vi "Complete Request.vi"(4 "WebSocket Handler":refnum<class "WebSocket Handler.lvclass">, 9 "Complete Handler Map":T1, 11 "Processing In":refnum<class "Processing.lvclass">) -> (3 "HTTP Server.lvlib:Processing":refnum<class "Processing.lvclass">)   [LabVIEW 2020, in "HTTP Server.lvlib" / "Server.lvclass"]
uses:
  Server.lvclass
  Processing/Processing.lvclass
  Complete Handler Map.ctl
  Priority.ctl
  Complete Handler/Complete Handler.lvclass
  WebSocket Handler/WebSocket Handler.lvclass
  C:/dev/lv20CE/relink/lv-http-server/HTTP Server/Handler/Handler.lvclass
  C:/dev/lv20CE/relink/lv-http-server/HTTP Server/Complete Handler/Complete Handler.lvclass
  Processing Step.ctl
  Processing/Processing.lvclass/Processing.ctl
  Handler/Handler.lvclass
  Server.lvclass/Server.ctl
  Session/Session.lvclass
  HTTP Server.lvlib
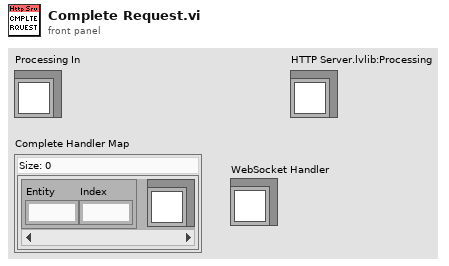
[diagram p1: front panel]
types:
  T1 = typedef "HTTP Server.lvlib/Complete Handler Map.ctl" = map{T2, refnum<class "Complete Handler.lvclass">}
  T2 = typedef "HTTP Server.lvlib/Priority.ctl" = cluster{"Entity":u16, "Index":u16}
  T3 = typedef "HTTP Server.lvlib/Processing Step.ctl" = enum16{"Connection", "Request", "Routing", "Controller Init", "Controller", "Response", "Complete", "Exception"}
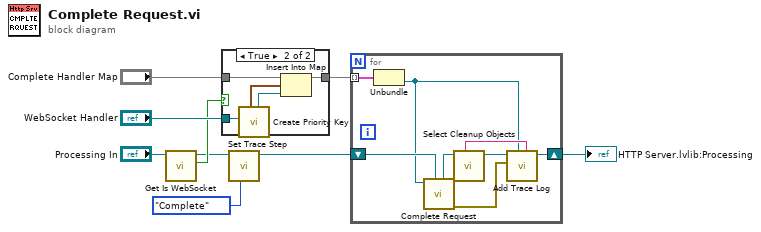
[diagram p0: block diagram]
diagram:
  n1 = call "Get Is WebSocket.vi"("Processing in"="Processing In") -> ("Is WebSocket"=w5:bool, "Processing out"=w4:refnum<class "Processing.lvclass">)  [unwired: 9 in]
  n2 = case shown="True" w5 {
    tunnel: "Complete Handler Map" -> [w10 w13]
    tunnel: "WebSocket Handler" -> [_ w11]
    tunnel: [w10 w12] -> w7
    frame False {
    }
    frame True {
      n3 = call "Create Priority Key.vi"("Handler In"=w11) -> ("Handler"=w14:refnum<class "WebSocket Handler.lvclass">, "Priority Key"=w15:T2)  [unwired: 8 in, 1 out]
      n4 = Insert Into Map(map in=w13, key=w15, value=w14) -> (map out=w12:T1)  [unwired: 2 out]
    }
  }
  n5 = call "Set Trace Step.vi"("Processing Step"=Processing_Step."Complete", "Processing in"=w4) -> ("Processing out"=w3:refnum<class "Processing.lvclass">)  [unwired: 9 in]
  n6 = for {
    tunnel: w7 -> [w23] mode=indexing
    shift-right: [w16] -> w2
    shift-left: w3 -> [w22]
    n7 = Unbundle(w23) -> ("Handler"=w17:refnum<class "Complete Handler.lvclass">)  [unwired: 1 out]
    n8 = call-dynamic "Complete Request.vi"("Processing In"=w22, "Complete Handler in"=w17) -> ("error out"=w19:errorcluster, "Processing"=w21:refnum<class "Processing.lvclass">)  [unwired: 8 in]
    n9 = call "Select Cleanup Objects.vi"("HTTP Server.lvlib:Processing"=w21) -> ("Updated Inputs"=w20:refnum<class "Processing.lvclass">, "Trace Message"=w18:string)  [unwired: 9 in]
    n10 = call "Add Trace Log.vi"("Info"=w18, "LabVIEW Object"=w17, "error in (no error)"=w19, "Processing in"=w20) -> ("Processing out"=w16:refnum<class "Processing.lvclass">)  [unwired: 6 in, 1 out]
  }
  "HTTP Server.lvlib:Processing" <- w2
